vi "Auto Detect_Programming Mode_Change property value.vi"(8 "error in (no error)":errorcluster, 10 "Slot Programming Mode":T1, 11 "Refnum in":refnum<k20>) -> (0 "error out":errorcluster, 3 "Refnum out":refnum<k20>)   [LabVIEW 2017, in "Scan Engine Custom Device.lvlib"]
doc: "Apply new \"Slot Prgramming Mode\" property value."
uses:
  Scan Engine Custom Device.lvlib
  Type Defs/Slot Programming Mode.ctl
  <vilib>/nisyscfg/Save Changes (Hardware).vi
  <resource>/objmgr/motionsysapi.rc
  <vilib>/nisyscfg/nisyscfg.lvlib
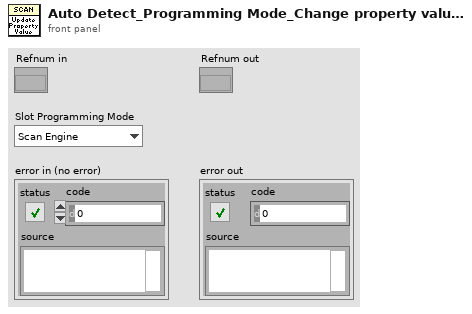
[diagram p1: front panel]
types:
  T1 = typedef "Scan Engine Custom Device.lvlib/Slot Programming Mode.ctl" = enum16{"Scan Engine", "LabVIEW FPGA", "NI-DAQmx", "Don't Modify"}
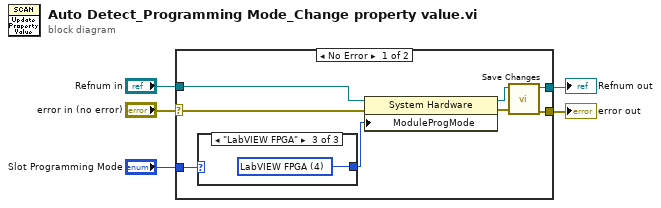
[diagram p0: block diagram]
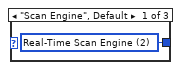
[diagram p2: hidden frame]
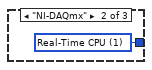
[diagram p3: hidden frame]
diagram:
  n1 = case shown="No Error" "error in (no error)" {
    selector: "error in (no error)" -> [w6 w17]
    tunnel: "Slot Programming Mode" -> [w12 _]
    tunnel: [w11 w18] -> w4
    tunnel: [w10 w17] -> w3
    tunnel: "Refnum in" -> [w7 w18]
    frame No Error {
      n2 = case shown="\"LabVIEW FPGA\"" w12 {
        tunnel: [w14 w15 w16] -> w13
        frame "Scan Engine", Default {
          w14 = u32 2 items=["None"=0, "Real-Time CPU"=1, "Real-Time Scan Engine"=2, "LabVIEW FPGA"=4] ("Devices & Chassis:Bus Specific:cRIO Module Programming Mode")
        }
        frame "NI-DAQmx" {
          w15 = u32 1 items=["None"=0, "Real-Time CPU"=1, "Real-Time Scan Engine"=2, "LabVIEW FPGA"=4] ("Devices & Chassis:Bus Specific:cRIO Module Programming Mode")
        }
        frame "LabVIEW FPGA" {
          w16 = u32 4 items=["None"=0, "Real-Time CPU"=1, "Real-Time Scan Engine"=2, "LabVIEW FPGA"=4] ("Devices & Chassis:Bus Specific:cRIO Module Programming Mode")
        }
      }
      n3 = property class="System Hardware"(reference=w7, error in=w6, "ModuleProgMode"=w13) -> (reference out=w9:refnum<k20>, error out=w8:errorcluster)
      n4 = call-poly <vilib>:"Save Changes.vi"("error in (no error)"=w8, "Resource in"=w9) -> ("error out"=w10:errorcluster, "Resource out"=w11:refnum<k20>)  [unwired: 6 in, 2 out]
    }
    frame Error {
    }
  }
  "Refnum out" <- w4
  "error out" <- w3
